vi "Build Tree Metadata.vi"(9 "Write Channel Data in":T4, 10 "Read Channel Data in":T4, 11 "Sh Var Data Array":T2[](array[typedef])) -> (1 "Write Channel Data out":T4, 2 "Read Channel Data out":T4, 3 "List Out":T1)   [LabVIEW 2012, in "Shared Variable Custom Device.lvlib"]
uses:
  Shared Variable Custom Device.lvlib
  Tree Data.ctl
  <vilib>/Utility/VariantDataType/Type.ctl
  Existing Channel Data.ctl
  List Cluster.ctl
  Shared/Shared Variable Globals.vi
  <vilib>/Utility/VariantDataType/VariantType.lvlib
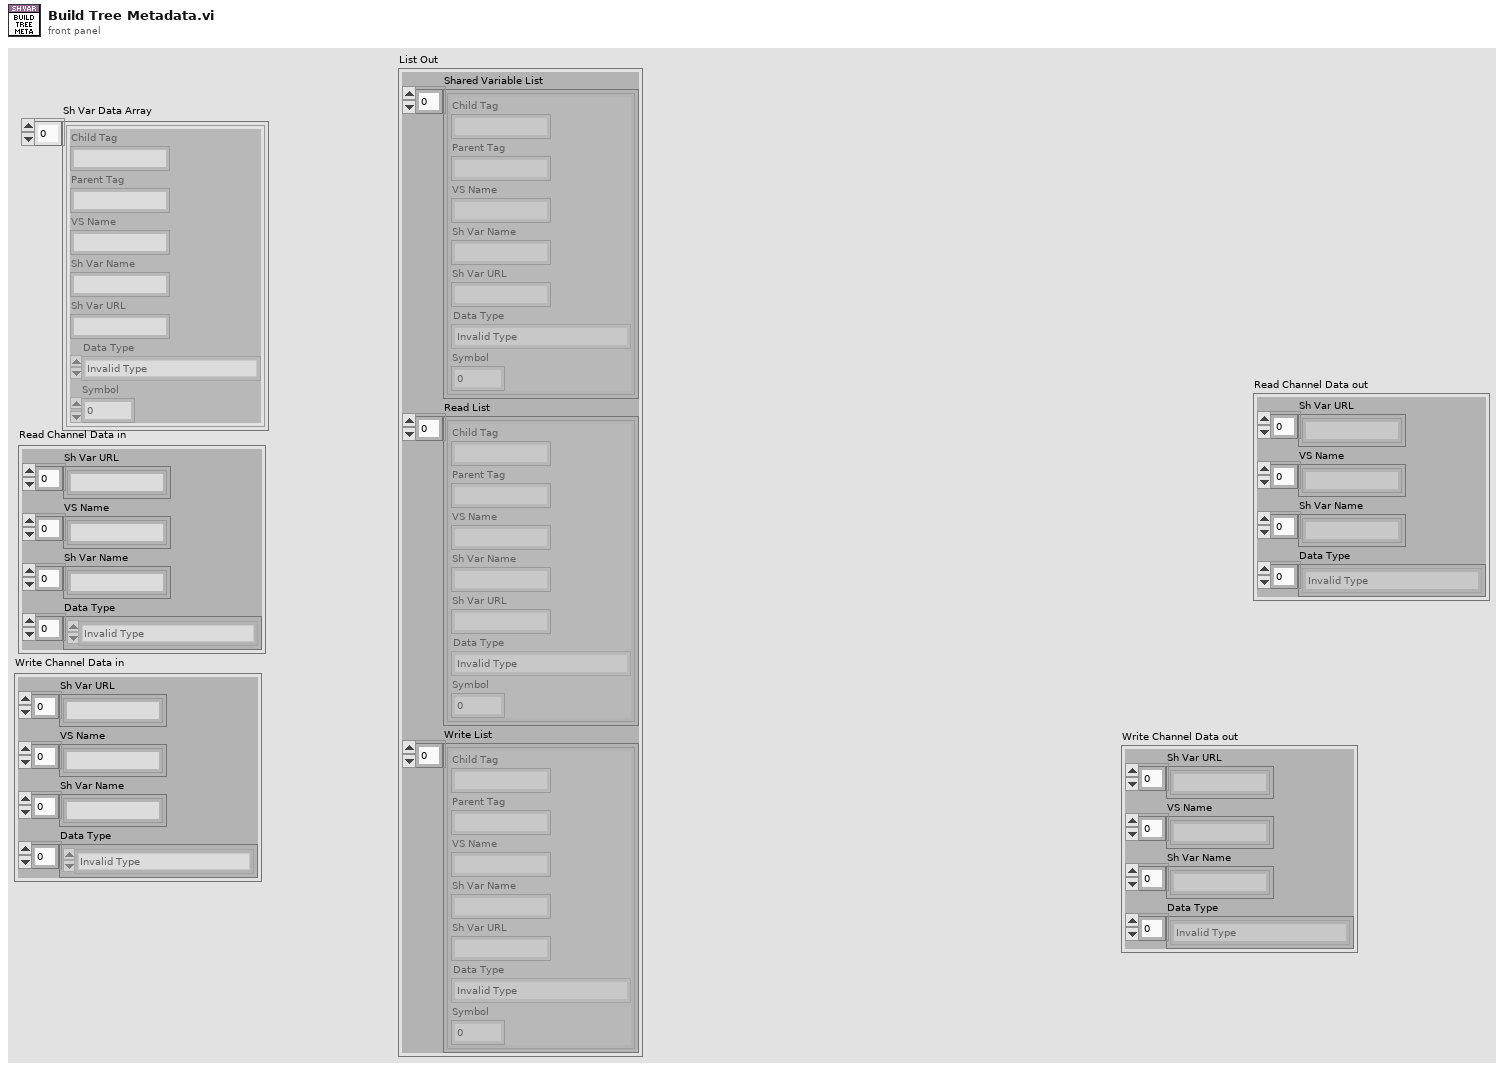
[diagram p1: front panel]
types:
  T1 = typedef "Shared Variable Custom Device.lvlib/List Cluster.ctl" = cluster{"Shared Variable List":T2[], "Read List":T2[], "Write List":T2[]}
  T2 = typedef "Shared Variable Custom Device.lvlib/Tree Data.ctl" = cluster{"Child Tag":string, "Parent Tag":string, "VS Name":string, "Sh Var Name":string, "Sh Var URL":string, "Data Type":T3, "Symbol":i32}
  T3 = typedef "VariantType.lvlib/Type.ctl" = enum8{"Invalid Type", "Void", "I8", "I16", "I32", "I64", "U8", "U16", "U32", "U64", "Single Float", "Double Float", "Extended Float", "Single Complex", "Double Complex", "Extended Complex", "Enum U8", "Enum U16", "Enum U32", "Enum U64", "Single Float With Unit", "Double Float With Unit", "Extended Float With Unit", "Single Complex with Unit", "Double Complex with Unit", "Extended Complex with Unit", "Boolean", "String", "Path", "Picture", "Tag", "Array", "Cluster", "Variant", "LV Variant", "Waveform", "Timestamp", "Digital Waveform", "Digital Data", "ExpressData", "Refnum", "External Data", "VI", "Poly VI", "LabVIEW Class Instance", "Fixed Point"}
  T4 = typedef "Shared Variable Custom Device.lvlib/Existing Channel Data.ctl" = cluster{"Sh Var URL":string[], "VS Name":string[], "Sh Var Name":string[], "Data Type":T3[]}
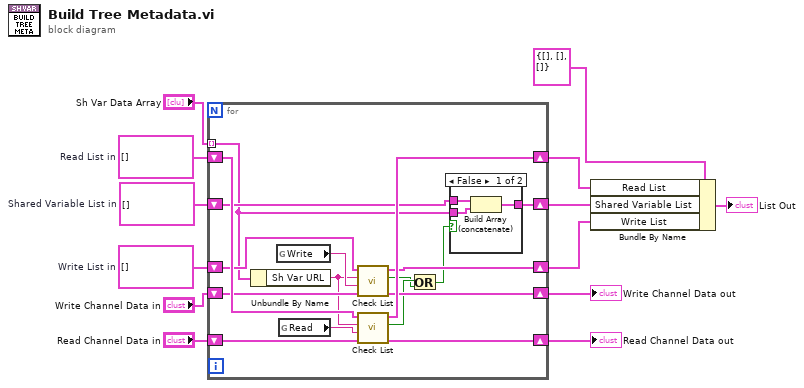
[diagram p0: block diagram]
diagram:
  w11 = T2[] []  # Read List in
  w12 = T2[] []  # Write List in
  w13 = T2[] []  # Shared Variable List in
  n1 = for {
    shift-right: [w16] -> w4
    shift-left: w13 -> [w17]
    shift-right: [w24] -> w3
    shift-left: w12 -> [w25]
    shift-right: [w26] -> w5
    shift-left: w11 -> [w30]
    tunnel: "Sh Var Data Array" -> [w14] mode=indexing
    shift-right: [w27] -> w7
    shift-left: "Read Channel Data in" -> [w28]
    shift-right: [w21] -> w6
    shift-left: "Write Channel Data in" -> [w22]
    n2 = Unbundle By Name(w14) -> ("Sh Var URL"=w15:string)
    n3 = global read "Shared Variable Globals.vi" "Write"() -> (w23:string)
    n4 = global read "Shared Variable Globals.vi" "Read"() -> (w29:string)
    n5 = call "Check List.vi"("Channel Data in"=w22, "Parent Tag"=w23, "Sh Var URL"=w15, "List in"=w25) -> ("Channel Data out"=w21:T4, "Found?"=w19:bool, "List out"=w24:T2[])  [unwired: 5 in]
    n6 = call "Check List.vi"("Channel Data in"=w28, "Parent Tag"=w29, "Sh Var URL"=w15, "List in"=w30) -> ("Channel Data out"=w27:T4, "Found?"=w20:bool, "List out"=w26:T2[])  [unwired: 5 in]
    n7 = Or(x=w20, y=w19) -> (x .or. y?=w18:bool)
    n8 = case shown="False" w18 {
      tunnel: w17 -> [w33 w34]
      tunnel: [w32 w34] -> w16
      tunnel: w14 -> [w31 _]
      frame False {
        n9 = Build Array (concatenate)(w33, w31) -> (w32:T2[])
      }
      frame True {
      }
    }
  }
  "Read Channel Data out" <- w7
  "Write Channel Data out" <- w6
  n10 = Bundle By Name(cluster=T1 {"Shared Variable List"=[], "Read List"=[], "Write List"=[]} ("List Out"), "Read List"=w5, "Shared Variable List"=w4, "Write List"=w3) -> (→"List Out":T1)
